vi "Execute.vi"(8 "error in (no error)":errorcluster, 11 "Start Pre-Soak in":refnum<class "Wait.lvclass">) -> (0 "error out":errorcluster, 3 "Start Pre-Soak out":refnum<class "Wait.lvclass">)   [LabVIEW 2019, in "Wait.lvclass"]
uses:
  <vilib>/gpm_packages/@cs/Car-wash/Source/Process Steps/Wait/Wait.lvclass
  C:/Program Files/National Instruments/LabVIEW 2019/vi.lib/ActorFramework/Actor/Actor.lvclass
  <vilib>/gpm_packages/@cs/Car-wash/Source/Process Steps/Wait Messages/Evaluate Wait Msg/Evaluate Wait Msg.lvclass
  C:/Program Files/National Instruments/LabVIEW 2019/vi.lib/ActorFramework/Message/Message.lvclass
  <vilib>/ActorFramework/Actor/Actor.lvclass/Actor.ctl
  <vilib>/ActorFramework/Message Enqueuer/Message Enqueuer.lvclass/Message Enqueuer.ctl
  <vilib>/gpm_packages/@cs/Car-wash/Source/Process Steps/Wait/Wait.lvclass/Wait.ctl
  <vilib>/ActorFramework/Message Enqueuer/Init from Existing Queue.vi
  <vilib>/ActorFramework/Message Enqueuer/Message Enqueuer.lvclass
  <vilib>/ActorFramework/Actor/Actor.lvclass
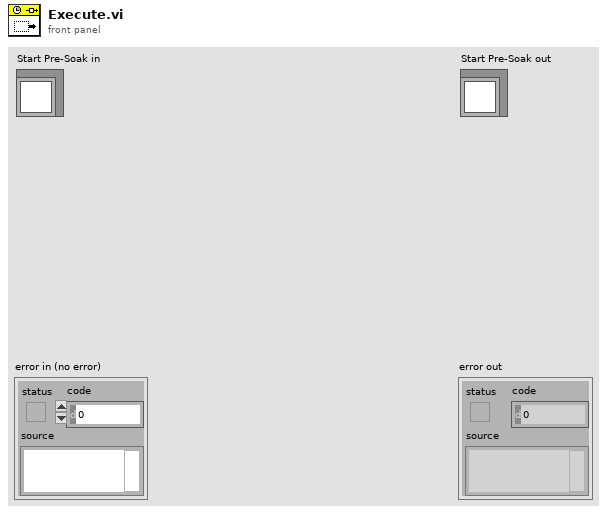
[diagram p1: front panel]
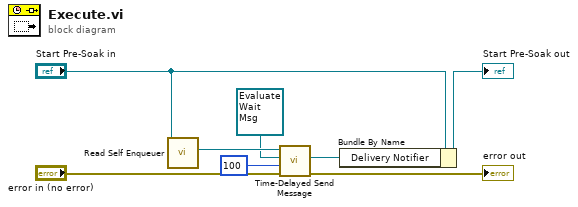
[diagram p0: block diagram]
diagram:
  n1 = call <vilib>:"Read Self Enqueuer.vi"("Actor"="Start Pre-Soak in") -> ("Self Enqueuer"=w8:refnum<class "Message Enqueuer.lvclass">)  [unwired: 10 in]
  n2 = call <vilib>:"Time-Delayed Send Message.vi"("error in (no error)"="error in (no error)", "Milliseconds To Wait"=100, "Message"=refnum<class "Evaluate Wait Msg.lvclass"> refnum ("Evaluate Wait Msg.lvclass"), "Message Enqueuer"=w8) -> ("error out"=→"error out":errorcluster, "Delivery Notifier"=w1:refnum<notifier>)  [unwired: 6 in]
  n3 = Bundle By Name(cluster="Start Pre-Soak in", "Delivery Notifier"=w1) -> (→"Start Pre-Soak out":refnum<class "Wait.lvclass">)
